vi "FTW-JSON-ReconstructFromBuffer.vi"(0 "JSON Object":refnum<class "FTW-JSON.lvclass">, 5 "JSON String (UTF-8)":string, 11 "error in":errorcluster) -> (4 "JSON Object":refnum<class "FTW-JSON.lvclass">, 15 "error out":errorcluster)   [LabVIEW 2013, in "FTW-JSON.lvclass"]
uses:
  FTW-JSON.lvclass
  FTW-JSON.lvclass/FTW-JSON.ctl
panel:
  # "Inputs"
  # "Outputs"
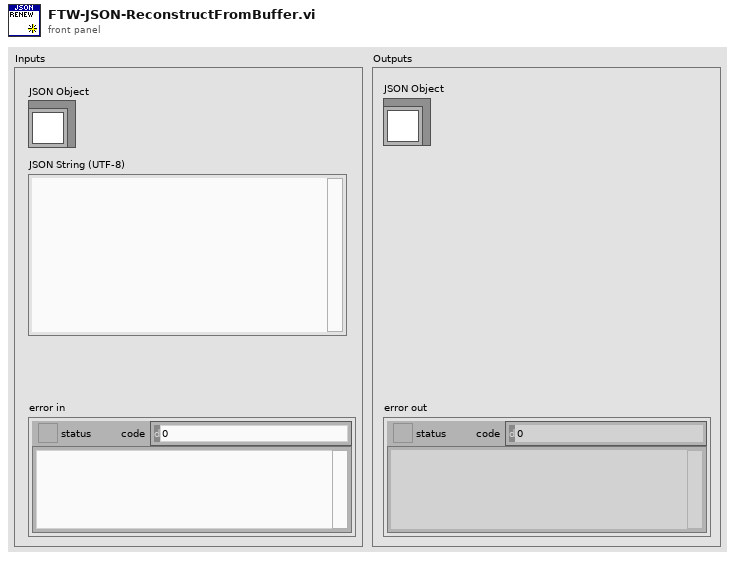
[diagram p1: front panel]
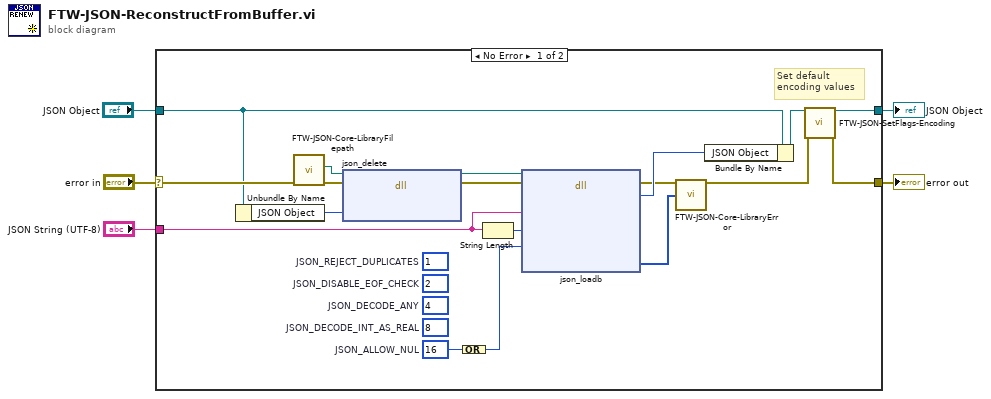
[diagram p0: block diagram]
diagram:
  n1 = case shown="No Error" "error in" {
    selector: "error in" -> [w23 w25]
    tunnel: [w12 w25] -> w5
    tunnel: [w14 w24] -> w3
    tunnel: "JSON Object" -> [w7 w24]
    tunnel: "JSON String (UTF-8)" -> [w19 _]
    frame No Error {
      w16 = u64 16  # JSON_ALLOW_NUL
      (unwired) u64 8  # JSON_DECODE_INT_AS_REAL
      (unwired) u64 4  # JSON_DECODE_ANY
      (unwired) u64 2  # JSON_DISABLE_EOF_CHECK
      (unwired) u64 1  # JSON_REJECT_DUPLICATES
      # "Set default\nencoding values"
      n2 = Unbundle By Name(w7) -> ("JSON Object"=w6:i64)
      n3 = call "FTW-JSON-Core-LibraryFilepath.vi"("error in"=w23) -> ("error out"=w8:errorcluster, "JSON Library Filepath"=w11:path)  [unwired: 9 in]
      n4 = dll-call lib="?" fn="json_delete"(path in=w11, error in=w8, "JSON Object Pointer"=w6) -> (path out=w10:path, error out=w9:errorcluster)  [unwired: 3 in]
      n5 = Compound Arithmetic op=OR(w16) -> (w17:u64)
      n6 = String Length(string=w19) -> (length=w18:i32)
      n7 = dll-call lib="?" fn="json_loadb"(path in=w10, error in=w9, "JSON Buffer"=w19, "Buffer Size"=w18, "Flags"=w17) -> (error out=w21:errorcluster, "JSON Object Pointer"=w22:i64, "Error Structure"=w20:u8[])  [unwired: 5 in, 1 out]
      n8 = call "FTW-JSON-Core-LibraryError.vi"("error in"=w21, "Error Structure"=w20) -> ("error out"=w13:errorcluster)  [unwired: 13 in]
      n9 = Bundle By Name(cluster=w7, "JSON Object"=w22) -> (w15:refnum<class "FTW-JSON.lvclass">)
      n10 = call "FTW-JSON-SetFlags-Encoding.vi"("JSON Object"=w15, "error in"=w13) -> ("JSON Object out"=w14:refnum<class "FTW-JSON.lvclass">, "error out"=w12:errorcluster)  [unwired: 12 in]
    }
    frame Error {
    }
  }
  "error out" <- w5
  "JSON Object" <- w3
